vi "Check VISA Installed.vi"() -> (3 "VISA Installed?":bool)   [LabVIEW 2019]
uses:
  <vilib>/Utility/sysdir.llb/System Directory Type.ctl
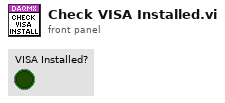
[diagram p1: front panel]
types:
  T1 = typedef "System Directory Type.ctl" = i32
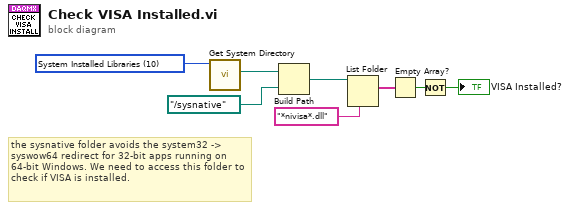
[diagram p0: block diagram]
diagram:
  w8 = T1 10 items=["User Home"=0, "User Desktop"=1, "User Documents"=2, "User Application Data"=3, "User Preferences"=4, "User Temporary"=5, "Public Documents"=6, "Public Application Data"=7, "Public Preferences"=8, "Public Cache"=13, "System Core Libraries"=9, "System Installed Libraries"=10, "Application Files"=11, "Boot Volume Root"=12] ("system directory type")
  # "the sysnative folder avoids the system32 -> syswow64 redirect for 32-bit apps running on 64-bit Windows. We need to access this folder to check if VISA is installed."
  n1 = call <vilib>:"Get System Directory.vi"("system directory type"=w8) -> ("system directory"=w5:path)  [unwired: 10 in]
  n2 = Build Path(base path=w5, name or relative path=path "../sysnative") -> (appended path=w4:path)
  n3 = List Folder(path=w4, pattern="*nivisa*.dll") -> (filenames=w3:string[])  [unwired: 2 in, 3 out]
  n4 = Empty Array?(array=w3) -> (empty?=w2:bool)
  n5 = Not(x=w2) -> (.not. x?=→"VISA Installed?":bool)
